vi "Retrieve Processes Spectrum.vi"(8 "error in (no error)":errorcluster) -> (0 "error out":errorcluster)   [LabVIEW 2017]
doc: "Retrieves the processed FFT spectrum and enqueues it for display or network transfer."
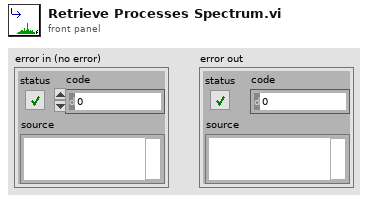
[diagram p1: front panel]
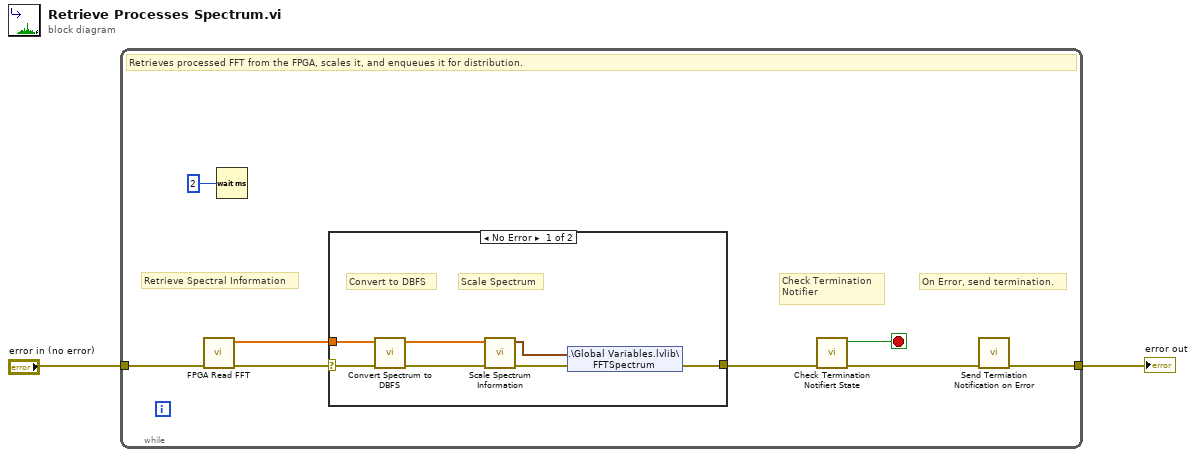
[diagram p0: block diagram]
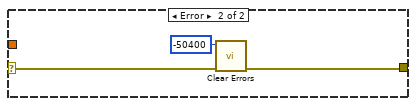
[diagram p2: hidden frame]
diagram:
  n1 = while {
    tunnel: "error in (no error)" -> [w10]
    tunnel: [w7] -> w1
    stop <- w8 stop-if-true
    # "On Error, send termination."
    # "Check Termination\nNotifier"
    # "Retrieve Spectral Information"
    # "Retrieves processed FFT from the FPGA, scales it, and enqueues it for distribution."
    n2 = call "FPGA Read FFT.vi"("error in (no error)"=w10) -> ("error out"=w4:errorcluster, "Spectral Information"=w3:dbl[])  [unwired: 9 in]
    n3 = Wait (ms)(milliseconds to wait=u32 2) -> ()  [unwired: 1 out]
    n4 = case shown="No Error" w4 {
      selector: w4 -> [w16 w19]
      tunnel: w3 -> [w17 _]
      tunnel: [w14 w18] -> w9
      frame No Error {
        # "Scale Spectrum"
        # "Convert to DBFS"
        n5 = call "Convert Spectrum to DBFS.vi"("error in (no error)"=w16, "Spectral Information"=w17) -> ("error out"=w15:errorcluster, "Spectral Information Out (DBFS)"=w11:dbl[])  [unwired: 8 in]
        n6 = call "Scale Spectrum Information.vi"("error in (no error)"=w15, "Spectral Information (DBFS)"=w11) -> ("error out"=w13:errorcluster, "Spectral Waveform"=w12:waveform(dbl))  [unwired: 8 in]
        n7 = shared-variable ".\\Global Variables.lvlib\\FFTSpectrum"(w12, error in=w13) -> (error out=w14:errorcluster)
      }
      frame Error {
        n8 = call <vilib>:"Clear Errors.vi"("error in (no error)"=w19, "specific error code to clear (0: all)"=-50400 ("y")) -> ("error out"=w18:errorcluster)  [unwired: 4 in, 1 out]
      }
    }
    n9 = call "Check Termination Notifiert State.vi"("error in (no error)"=w9) -> ("error out"=w6:errorcluster, "Termination Notifier State"=w8:bool)  [unwired: 9 in]
    n10 = call "Send Termiation Notification on Error.vi"("error in (no error)"=w6) -> ("error out"=w7:errorcluster)  [unwired: 10 in]
  }
  "error out" <- w1
